vi "Teleop.vi"(10 "Match Info":T1={"Autonomous Elapsed Seconds"=0.0, "TeleOp Elapsed Seconds"=0.0, "Disabled Elapsed Seconds"=0.0, "Visited Autonomous"=FALSE, "Visited TeleOp"=FALSE, "Visited Disabled"=FALSE, "Autonomous Settings"={"Autonomous Style"=enum."Independent", "VI Refnum"=refnum}}, 11 "Call Context":T2) -> ()   [LabVIEW 2011]
doc: "This VI is called for each TeleOp packet received from the DS where the robot is not disabled. It is often used to read from the joysticks and update I/O or to update setpoints for timed control loops. It should complete and return within 20 milliseconds or it may miss DS packets."
uses:
  <vilib>/Rock Robotics/WPI/DriverStation/WPI_DriverStationDerivedRobotMode.ctl
  <vilib>/Rock Robotics/WPI/DriverStation/WPI_DriverStationMatch Info.ctl
  <vilib>/Rock Robotics/WPI/Relay/WPI_RelayValue.ctl
  <vilib>/Rock Robotics/WPI/DriverStation/DriverStationLCD/WPI_DriverStationLCDLCDLine.ctl
  Robot Global Data.vi
panel:
  in  "LDrive0":dbl
  in  "Rdrive0":dbl=0.9
  in  "Rdrive2":dbl=0.6
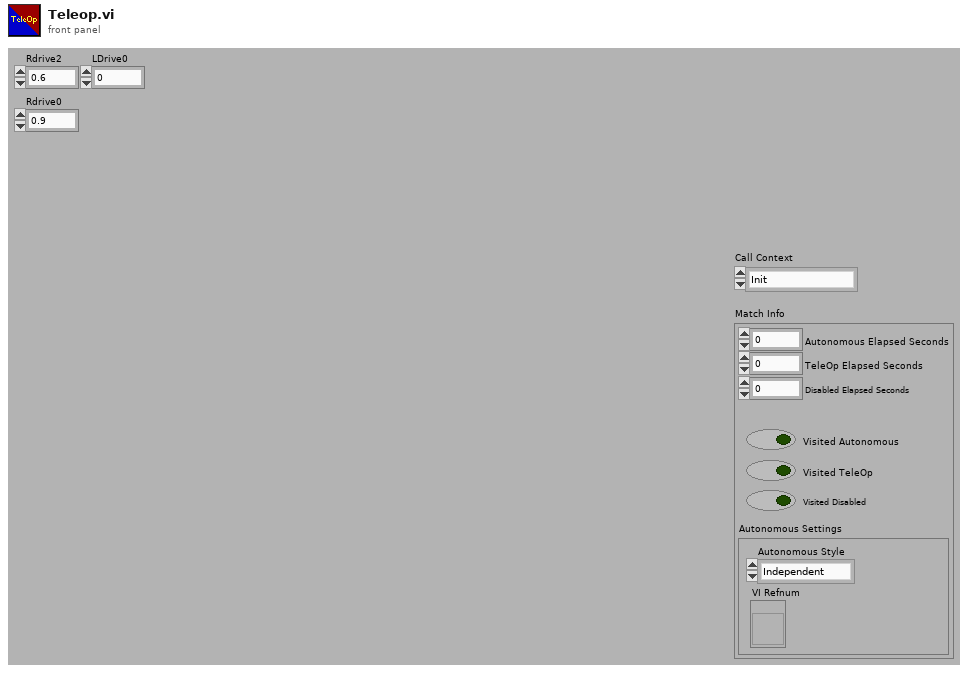
[diagram p1: front panel]
types:
  T1 = typedef "WPI_DriverStationMatch Info.ctl" = cluster{"Autonomous Elapsed Seconds":dbl, "TeleOp Elapsed Seconds":dbl, "Disabled Elapsed Seconds":dbl, "Visited Autonomous":bool, "Visited TeleOp":bool, "Visited Disabled":bool, "Autonomous Settings":cluster{"Autonomous Style":enum16{"Iterative", "Independent"}, "VI Refnum":refnum<vi>}}
  T2 = typedef "WPI_DriverStationDerivedRobotMode.ctl" = enum16{"Init", "Execute", "Stop"}
  T3 = typedef "WPI_RelayValue.ctl" = enum16{"Off", "On", "Forward", "Reverse"}
  T4 = typedef "WPI_JoystickDevRef.ctl" = cluster{"Device":T5}
  T5 = typedef "WPI_JoystickDeviceEnum.ctl" = enum16{"USB 1", "USB 2", "USB 3", "USB 4", "Kinect 1", "Kinect 2"}
  T6 = typedef "WPI_JoystickButtonState.ctl" = cluster{"Button 1":bool, "Button 2":bool, "Button 3":bool, "Button 4":bool, "Button 5":bool, "Button 6":bool, "Button 7":bool, "Button 8":bool, "Button 9":bool, "Button 10":bool, "Button 11":bool, "Button 12":bool}
  T7 = cluster{"axis 1 (x)":dbl, "axis 2 (y)":dbl, "axis 3 (throttle)":dbl, "axis 4":dbl, "axis 5":dbl, "axis 6":dbl}
  T8 = typedef "WPI_MotorControlDeviceRef.ctl" = cluster{"DeviceStatus":errorcluster, "Type":enum16{"PWM", "CAN"}, "PWM":cluster{"Digital Module":T9, "PWM Channel":T10, "DeadBand":T11}, "CAN":cluster{"Device Number":u8, "Control Mode":T12, "Semaphore":T13, "Max Vout":dbl}, "Invert":bool, "TransformRef":T14, "InvTransformRef":T14}
  T9 = typedef "FPGA_TypedefDigitalModule.ctl" = enum16{"Digital Module 1", "Digital Module 2"}
  T10 = typedef "FPGA_DIOPWMChannel.ctl" = enum8{"PWM 1", "PWM 2", "PWM 3", "PWM 4", "PWM 5", "PWM 6", "PWM 7", "PWM 8", "PWM 9", "PWM 10", "Invalid"}
  T11 = typedef "WPI_PWMDeadband.ctl" = cluster{"Name":string, "maxPositivePwm":i32, "minPositivePwm":i32, "centerPwm":i32, "maxNegativePwm":i32, "minNegativePwm":i32, "angularRange":u16}
  T12 = typedef "WPI_CANJaguar_ControlMode.ctl" = enum8{"Percent VBus", "Current", "Speed", "Position", "Voltage"}
  T13 = typedef "Semaphore RefNum" = refnum<k1>
  T14 = typedef "WPI_PWMTransform_ConPane.ctl" = refnum<vi>
  T15 = cluster{"Driver Station Digital Input (1-8)[0]":bool, "Driver Station Digital Input (1-8)[1]":bool, "Driver Station Digital Input (1-8)[2]":bool, "Driver Station Digital Input (1-8)[3]":bool, "Driver Station Digital Input (1-8)[4]":bool, "Driver Station Digital Input (1-8)[5]":bool, "Driver Station Digital Input (1-8)[6]":bool, "Driver Station Digital Input (1-8)[7]":bool, "Driver Station Digital Input (1-8)[8]":bool}
  T16 = typedef "WPI_RelayDevRef.ctl" = cluster{"DevStatus":errorcluster, "Relay Channel":T17, "Digital Module":T9, "Relay Direction":T18}
  T17 = typedef "FPGA_DIORelayChannel.ctl" = enum8{"Relay 1", "Relay 2", "Relay 3", "Relay 4", "Relay 5", "Relay 6", "Relay 7", "Relay 8", "Invalid"}
  T18 = typedef "WPI_RelayDirection.ctl" = enum16{"Both directions", "Forward only", "Reverse only"}
  T19 = typedef "WPI_DigitalInputDevRef.ctl" = cluster{"DevStatus":errorcluster, "DIO Channel":T20, "Digital Module":T9}
  T20 = typedef "FPGA_DIOChannel.ctl" = enum8{"DIO 1", "DIO 2", "DIO 3", "DIO 4", "DIO 5", "DIO 6", "DIO 7", "DIO 8", "DIO 9", "DIO 10", "DIO 11", "DIO 12", "DIO 13", "DIO 14", "Invalid"}
  T21 = typedef "WPI_EncoderDevRef.ctl" = cluster{"DevStatus":errorcluster, "EncoderIndex":T22, "CounterIndex":T23, "DistancePerCount":dbl, "Decoding Type":T24}
  T22 = typedef "FPGA_EncoderIdx.ctl" = enum8{"Enc 0", "Enc 1", "Enc 2", "Enc 3", "Invalid"}
  T23 = typedef "FPGA_CounterCtrSystemIndex.ctl" = enum8{"Ctr 0", "Ctr 1", "Ctr 2", "Ctr 3", "Ctr 4", "Ctr 5", "Ctr 6", "Ctr 7", "Invalid"}
  T24 = typedef "WPI_EncoderType.ctl" = enum16{"1x", "2x", "4x"}
  T25 = typedef "WPI_DriverStationLCDLCDLine.ctl" = enum16{"Main - Line 1", "User - Line 2", "User - Line 3", "User - Line 4", "User - Line 5", "User - Line 6"}
  T26 = typedef "WPI_ServoDeviceRef.ctl" = cluster{"DeviceStatus":errorcluster, "Digital Module":T9, "PWM Channel":T10, "DeadBand":T11}
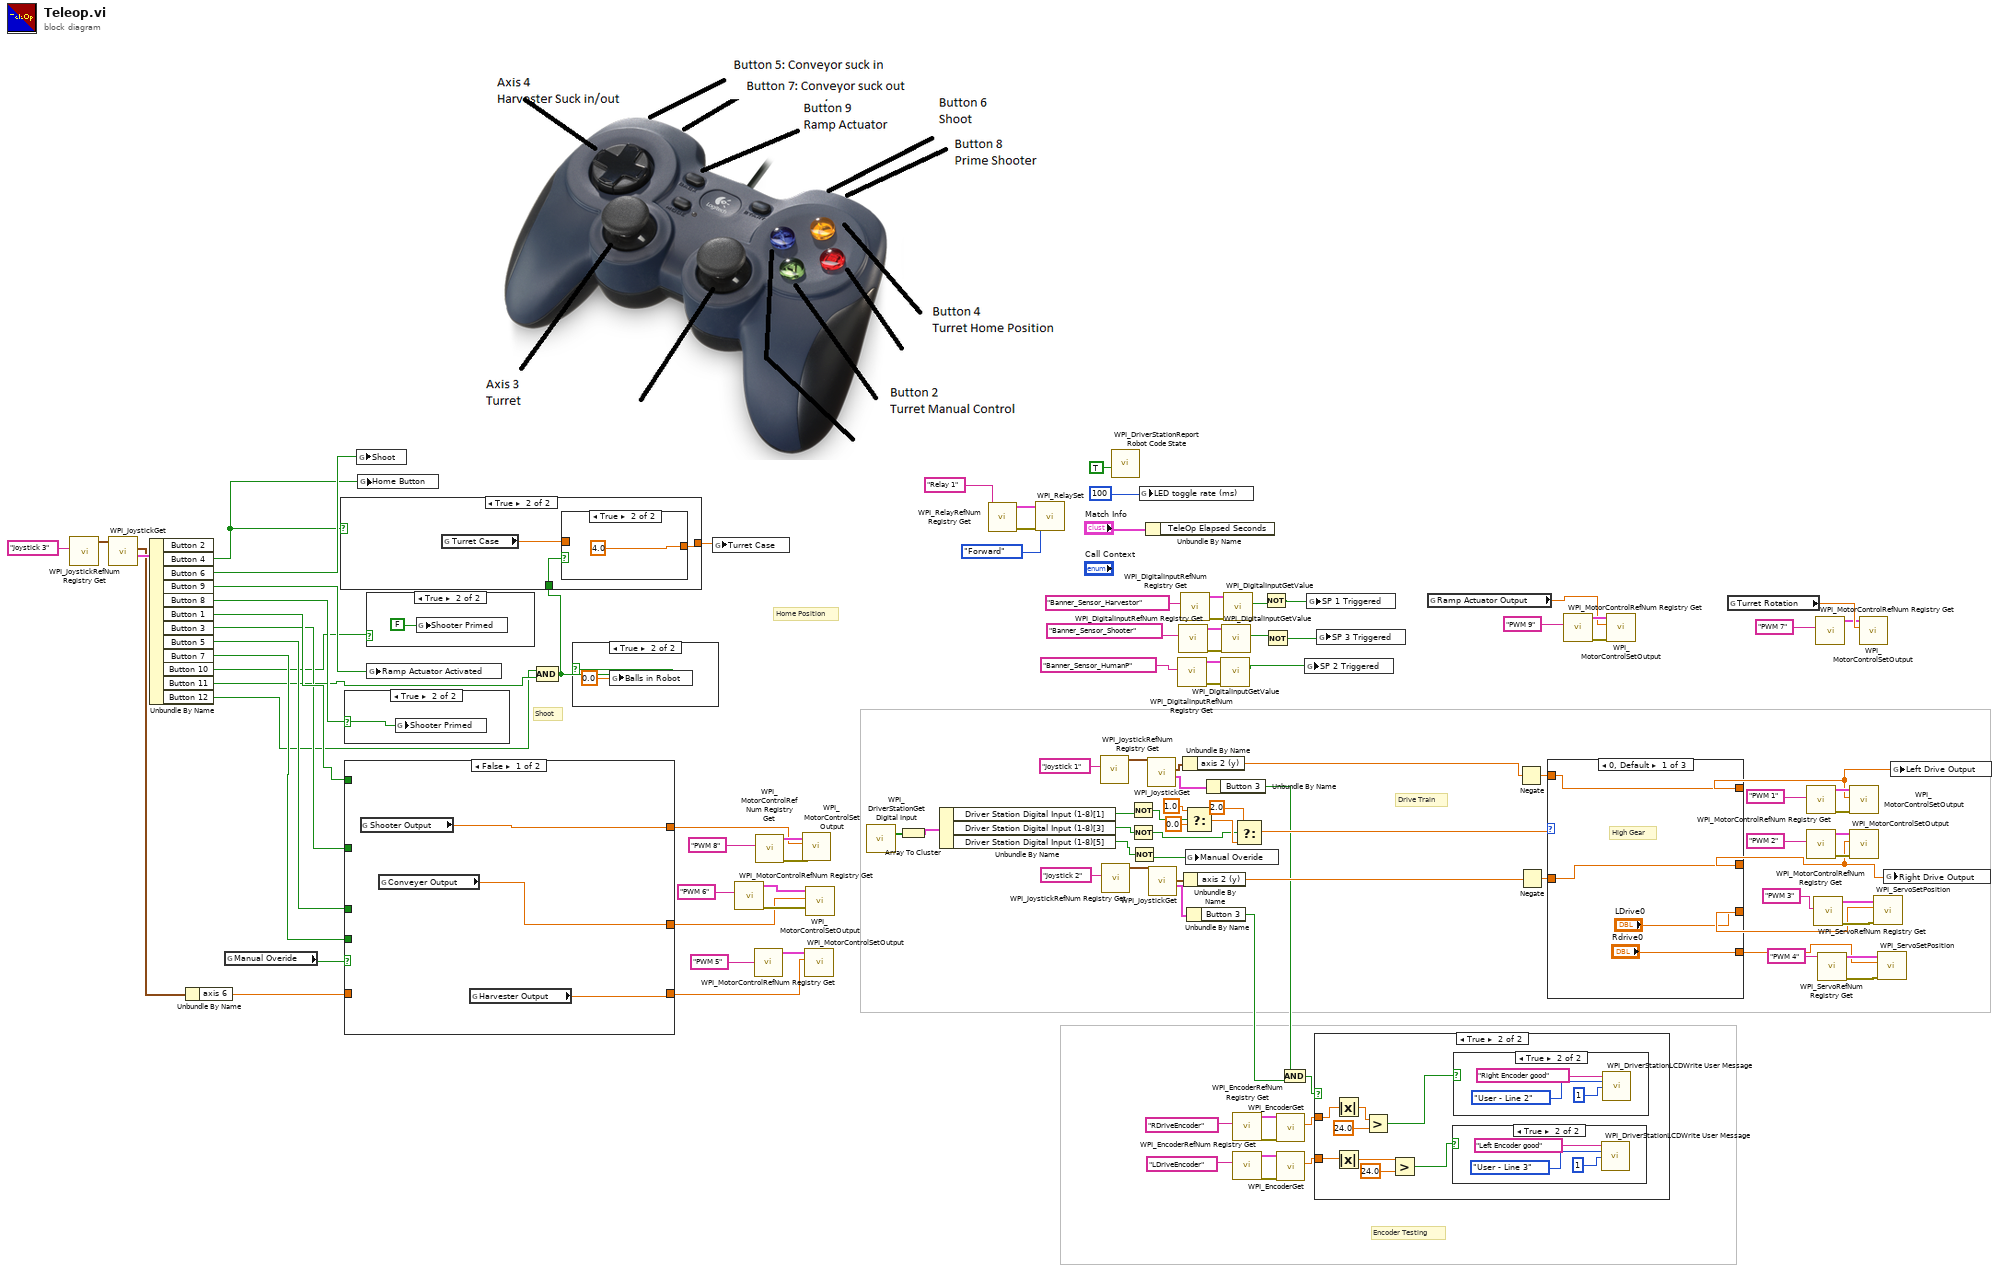
[diagram p0: block diagram]
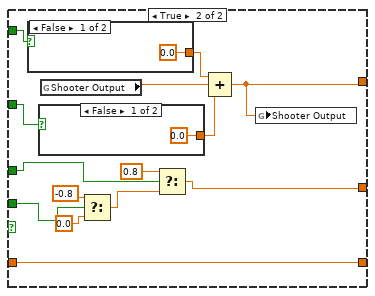
[diagram p7: hidden frame]
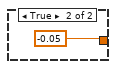
[diagram p8: hidden frame]
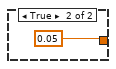
[diagram p9: hidden frame]
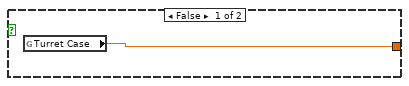
[diagram p11: hidden frame]
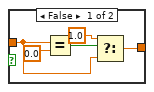
[diagram p12: hidden frame]
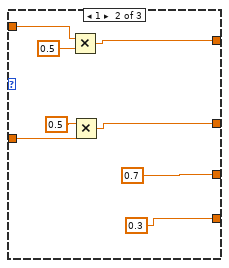
[diagram p13: hidden frame]
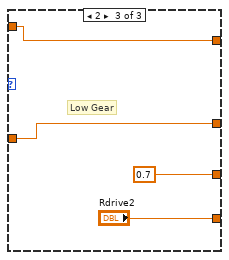
[diagram p14: hidden frame]
diagram:
  # "Encoder Testing"
  # "Shoot"
  # "Home Position"
  # "Drive Train"
  n1 = call <vilib>:"WPI_JoystickRefNum Registry Get.vi"("refnum name"="Joystick 3") -> ("JoystickDevRef"=w63:T4)  [unwired: 9 in, 1 out]
  n2 = call <vilib>:"WPI_JoystickGet.vi"("JoystickDevRef"=w63) -> ("Buttons"=w64:T6, "Axes"=w37:T7)  [unwired: 4 in, 1 out]
  n3 = Unbundle By Name(w64) -> ("Button 4"=w22:bool, "Button 6"=w62:bool, "Button 9"=w66:bool, "Button 8"=w38:bool, "Button 1"=w24:bool, "Button 3"=w23:bool, "Button 5"=w32:bool, "Button 7"=w31:bool, "Button 10"=w21:bool, "Button 11"=w20:bool, "Button 12"=w19:bool)  [unwired: 1 out]
  n4 = Unbundle By Name(w37) -> ("axis 6"=w17:dbl)
  n5 = global read "Robot Global Data.vi" "Manual Overide"() -> (w26:bool)
  n6 = case shown="True" w38 {
    selector: w38 -> [_ w111]
    frame False {
    }
    frame True {
      n7 = global write "Robot Global Data.vi" "Shooter Primed"(w111) -> ()
    }
  }
  n8 = case shown="False" w26 {
    tunnel: [w114 w116] -> w33
    tunnel: w24 -> [_ w121]
    tunnel: w23 -> [_ w120]
    tunnel: w32 -> [_ w123]
    tunnel: w31 -> [_ w124]
    tunnel: [w113 w122] -> w27
    tunnel: [w112 w115] -> w18
    tunnel: w17 -> [_ w115]
    frame False {
      n9 = global read "Robot Global Data.vi" "Shooter Output"() -> (w114:dbl)
      n10 = global read "Robot Global Data.vi" "Conveyer Output"() -> (w113:dbl)
      n11 = global read "Robot Global Data.vi" "Harvester Output"() -> (w112:dbl)
    }
    frame True {
      n12 = case shown="False" w121 {
        tunnel: [0.0 0.05] -> w119
        frame False {
        }
        frame True {
        }
      }
      n13 = case shown="False" w120 {
        tunnel: [0.0 -0.05] -> w118
        frame False {
        }
        frame True {
        }
      }
      n14 = global read "Robot Global Data.vi" "Shooter Output"() -> (w117:dbl)
      n15 = Select(t=-0.8, s=w124, f=0.0) -> (s? t:f=w128:dbl)
      n16 = Select(t=0.8, s=w123, f=w128) -> (s? t:f=w122:dbl)
      n17 = Compound Arithmetic op=ADD(w119, w117, w118) -> (w116:dbl)
      n18 = global write "Robot Global Data.vi" "Shooter Output"(w116) -> ()
    }
  }
  n19 = global write "Robot Global Data.vi" "Shoot"(w62) -> ()
  n20 = global write "Robot Global Data.vi" "Home Button"(w22) -> ()
  n21 = case shown="True" w21 {
    frame False {
    }
    frame True {
      n22 = global write "Robot Global Data.vi" "Shooter Primed"(FALSE ("Shooter Primed")) -> ()
    }
  }
  n23 = global write "Robot Global Data.vi" "Ramp Actuator Activated"(w66) -> ()
  n24 = Compound Arithmetic op=AND(w19, w20) -> (w16:bool)
  n25 = case shown="True" w22 {
    tunnel: [w134 w135] -> w15
    tunnel: w16 -> [_ w137]
    frame False {
      n26 = global read "Robot Global Data.vi" "Turret Case"() -> (w134:dbl)
    }
    frame True {
      n27 = global read "Robot Global Data.vi" "Turret Case"() -> (w136:dbl)
      n28 = case shown="True" w137 {
        tunnel: w136 -> [w139 _]
        tunnel: [w138 4.0 ("Turret Case")] -> w135
        frame False {
          n29 = Equal?(x=w139, y=0.0) -> (x = y?=w141:bool)
          n30 = Select(t=1.0, s=w141, f=w139) -> (s? t:f=w138:dbl)
        }
        frame True {
        }
      }
    }
  }
  n31 = case shown="True" w16 {
    frame False {
    }
    frame True {
      n32 = global write "Robot Global Data.vi" "Balls in Robot"(0.0 ("Balls in Robot")) -> ()
    }
  }
  n33 = global write "Robot Global Data.vi" "Turret Case"(w15) -> ()
  n34 = call <vilib>:"WPI_MotorControlRefNum Registry Get.vi"("refnum name"="PWM 6") -> ("error out"=w28:errorcluster, "MotorControlDevRef"=w29:T8)  [unwired: 9 in]
  n35 = call <vilib>:"WPI_MotorControlRefNum Registry Get.vi"("refnum name"="PWM 5") -> ("MotorControlDevRef"=w56:T8)  [unwired: 9 in, 1 out]
  n36 = call <vilib>:"WPI_MotorControlRefNum Registry Get.vi"("refnum name"="PWM 8") -> ("error out"=w40:errorcluster, "MotorControlDevRef"=w41:T8)  [unwired: 9 in]
  n37 = call <vilib>:"WPI_MotorControlSetOutput.vi"("error in (no error)"=w40, "Output"=w33, "MotorControlDevRef"=w41) -> ()  [unwired: 7 in, 2 out]
  n38 = call <vilib>:"WPI_MotorControlSetOutput.vi"("Output"=w18, "MotorControlDevRef"=w56) -> ()  [unwired: 8 in, 2 out]
  n39 = call <vilib>:"WPI_MotorControlSetOutput.vi"("error in (no error)"=w28, "Output"=w27, "MotorControlDevRef"=w29) -> ()  [unwired: 7 in, 2 out]
  n40 = call <vilib>:"WPI_DriverStationGet Digital Input.vi"() -> ("Driver Station Digital Input (1-8)"=w85:bool[])  [unwired: 11 in]
  n41 = Array To Cluster(array=w85) -> (cluster=w107:T15)
  n42 = Unbundle By Name(w107) -> ("Driver Station Digital Input (1-8)[1]"=w88:bool, "Driver Station Digital Input (1-8)[3]"=w87:bool, "Driver Station Digital Input (1-8)[5]"=w34:bool)
  n43 = call <vilib>:"WPI_RelayRefNum Registry Get.vi"("refnum name"="Relay 1") -> ("error out"=w60:errorcluster, "RelayDevRef"=w61:T16)  [unwired: 9 in]
  n44 = call <vilib>:"WPI_RelaySet.vi"("error in (no error)"=w60, "RelayValue"=WPI_RelayValue."Forward", "RelayDevRef"=w61) -> ()  [unwired: 7 in, 2 out]
  n45 = call <vilib>:"WPI_JoystickRefNum Registry Get.vi"("refnum name"="Joystick 1") -> ("JoystickDevRef"=w100:T4)  [unwired: 9 in, 1 out]
  n46 = call <vilib>:"WPI_JoystickRefNum Registry Get.vi"("refnum name"="Joystick 2") -> ("JoystickDevRef"=w98:T4)  [unwired: 9 in, 1 out]
  n47 = call <vilib>:"WPI_DriverStationReport Robot Code State.vi"("TeleOp"=TRUE ("Autonomous")) -> ()  [unwired: 10 in, 1 out]
  n48 = Not(x=w88) -> (.not. x?=w86:bool)
  n49 = Not(x=w87) -> (.not. x?=w36:bool)
  n50 = Not(x=w34) -> (.not. x?=w35:bool)
  n51 = global write "Robot Global Data.vi" "LED toggle rate (ms)"(u32 100 ("LED ms toggle rate")) -> ()
  n52 = Unbundle By Name("Match Info") -> ()  [unwired: 1 out]
  n53 = call <vilib>:"WPI_JoystickGet.vi"("JoystickDevRef"=w100) -> ("Buttons"=w12:T6, "Axes"=w13:T7)  [unwired: 4 in, 1 out]
  n54 = call <vilib>:"WPI_JoystickGet.vi"("JoystickDevRef"=w98) -> ("Buttons"=w14:T6, "Axes"=w99:T7)  [unwired: 4 in, 1 out]
  n55 = call <vilib>:"WPI_DigitalInputRefNum Registry Get.vi"("refnum name"="Banner_Sensor_HumanP") -> ("error out"=w51:errorcluster, "DigitalInputDevRef"=w50:T19)  [unwired: 9 in]
  n56 = call <vilib>:"WPI_DigitalInputRefNum Registry Get.vi"("refnum name"="Banner_Sensor_Shooter") -> ("error out"=w52:errorcluster, "DigitalInputDevRef"=w53:T19)  [unwired: 9 in]
  n57 = call <vilib>:"WPI_DigitalInputRefNum Registry Get.vi"("refnum name"="Banner_Sensor_Harvestor") -> ("error out"=w55:errorcluster, "DigitalInputDevRef"=w54:T19)  [unwired: 9 in]
  n58 = Unbundle By Name(w13) -> ("axis 2 (y)"=w84:dbl)
  n59 = Unbundle By Name(w99) -> ("axis 2 (y)"=w82:dbl)
  n60 = Select(t=1.0, s=w86, f=0.0 ("t")) -> (s? t:f=w104:dbl)
  n61 = global write "Robot Global Data.vi" "Manual Overide"(w35) -> ()
  n62 = Unbundle By Name(w14) -> ("Button 3"=w10:bool)
  n63 = Unbundle By Name(w12) -> ("Button 3"=w11:bool)
  n64 = call <vilib>:"WPI_DigitalInputGetValue.vi"("error in (no error)"=w51, "DigitalInputDevRef"=w50) -> ("Value"=w46:bool)  [unwired: 7 in, 2 out]
  n65 = call <vilib>:"WPI_DigitalInputGetValue.vi"("error in (no error)"=w52, "DigitalInputDevRef"=w53) -> ("Value"=w45:bool)  [unwired: 7 in, 2 out]
  n66 = call <vilib>:"WPI_DigitalInputGetValue.vi"("error in (no error)"=w55, "DigitalInputDevRef"=w54) -> ("Value"=w43:bool)  [unwired: 7 in, 2 out]
  n67 = call <vilib>:"WPI_EncoderRefNum Registry Get.vi"("refnum name"="RDriveEncoder") -> ("error out"=w6:errorcluster, "EncoderDevRef"=w7:T21)  [unwired: 9 in]
  n68 = call <vilib>:"WPI_EncoderRefNum Registry Get.vi"("refnum name"="LDriveEncoder") -> ("error out"=w5:errorcluster, "EncoderDevRef"=w4:T21)  [unwired: 9 in]
  n69 = Select(t=2.0, s=w36, f=w104) -> (s? t:f=w102:dbl)
  n70 = Not(x=w43) -> (.not. x?=w42:bool)
  n71 = Not(x=w45) -> (.not. x?=w44:bool)
  n72 = call <vilib>:"WPI_EncoderGet.vi"("error in (no error)"=w6, "EncoderDevRef"=w7) -> ("Distance"=w2:dbl)  [unwired: 4 in, 5 out]
  n73 = call <vilib>:"WPI_EncoderGet.vi"("error in (no error)"=w5, "EncoderDevRef"=w4) -> ("Distance"=w1:dbl)  [unwired: 4 in, 5 out]
  n74 = And(x=w11, y=w10) -> (x .and. y?=w9:bool)
  n75 = global write "Robot Global Data.vi" "SP 2 Triggered"(w46) -> ()
  n76 = global write "Robot Global Data.vi" "SP 1 Triggered"(w42) -> ()
  n77 = case shown="True" w9 {
    tunnel: w2 -> [_ w147]
    tunnel: w1 -> [_ w146]
    frame False {
    }
    frame True {
      n78 = Absolute Value(x=w147) -> (abs(x)=w148:dbl)
      n79 = Absolute Value(x=w146) -> (abs(x)=w145:dbl)
      n80 = Greater?(x=w148, y=24.0) -> (0:w151:bool)
      n81 = Greater?(x=w145, y=24.0) -> (0:w149:bool)
      n82 = case shown="True" w149 {
        frame False {
        }
        frame True {
          n83 = call <vilib>:"WPI_DriverStationLCDWrite User Message.vi"("line text"="Left Encoder good", "line"=WPI_DriverStationLCDLCDLine."User - Line 3", "starting column"=i8 1) -> ()  [unwired: 2 in, 11 out]
        }
      }
      n84 = case shown="True" w151 {
        frame False {
        }
        frame True {
          n85 = call <vilib>:"WPI_DriverStationLCDWrite User Message.vi"("line text"="Right Encoder good", "line"=WPI_DriverStationLCDLCDLine."User - Line 2", "starting column"=i8 1) -> ()  [unwired: 2 in, 11 out]
        }
      }
    }
  }
  n86 = global write "Robot Global Data.vi" "SP 3 Triggered"(w44) -> ()
  n87 = global read "Robot Global Data.vi" "Ramp Actuator Output"() -> (w25:dbl)
  n88 = Negate(x=w84) -> (-x=w83:dbl)
  n89 = Negate(x=w82) -> (-x=w81:dbl)
  n90 = case shown="0, Default" w102 {
    tunnel: w81 -> [w162 w167 w174]
    tunnel: [w162 w168 w174] -> w73
    tunnel: [w161 w169 w173] -> w74
    tunnel: ["LDrive0" 0.7 0.7] -> w90
    tunnel: ["Rdrive0" 0.3 ("LeftShifter_Pos") "Rdrive2"] -> w89
    tunnel: w83 -> [w161 w165 w173]
    frame 0, Default {
      # "High Gear"
    }
    frame 1 {
      n91 = Multiply(x=w165, y=0.5) -> (x*y=w169:dbl)
      n92 = Multiply(x=0.5 ("y"), y=w167) -> (x*y=w168:dbl)
    }
    frame 2 {
      # "Low Gear"
    }
  }
  n93 = call <vilib>:"WPI_MotorControlRefNum Registry Get.vi"("refnum name"="PWM 9") -> ("error out"=w71:errorcluster, "MotorControlDevRef"=w70:T8)  [unwired: 9 in]
  n94 = call <vilib>:"WPI_MotorControlSetOutput.vi"("error in (no error)"=w71, "Output"=w25, "MotorControlDevRef"=w70) -> ()  [unwired: 7 in, 2 out]
  n95 = global read "Robot Global Data.vi" "Turret Rotation"() -> (w69:dbl)
  n96 = call <vilib>:"WPI_MotorControlRefNum Registry Get.vi"("refnum name"="PWM 1") -> ("error out"=w78:errorcluster, "MotorControlDevRef"=w80:T8)  [unwired: 9 in]
  n97 = call <vilib>:"WPI_MotorControlRefNum Registry Get.vi"("refnum name"="PWM 2") -> ("error out"=w77:errorcluster, "MotorControlDevRef"=w76:T8)  [unwired: 9 in]
  n98 = call <vilib>:"WPI_ServoRefNum Registry Get.vi"("refnum name"="PWM 3") -> ("error out"=w94:errorcluster, "ServoDeviceRef"=w95:T26)  [unwired: 9 in]
  n99 = call <vilib>:"WPI_MotorControlRefNum Registry Get.vi"("refnum name"="PWM 7") -> ("MotorControlDevRef"=w67:T8)  [unwired: 9 in, 1 out]
  n100 = call <vilib>:"WPI_ServoRefNum Registry Get.vi"("refnum name"="PWM 4") -> ("error out"=w93:errorcluster, "ServoDeviceRef"=w92:T26)  [unwired: 9 in]
  n101 = call <vilib>:"WPI_MotorControlSetOutput.vi"("error in (no error)"=w78, "Output"=w74, "MotorControlDevRef"=w80) -> ()  [unwired: 7 in, 2 out]
  n102 = call <vilib>:"WPI_MotorControlSetOutput.vi"("error in (no error)"=w77, "Output"=w73, "MotorControlDevRef"=w76) -> ()  [unwired: 7 in, 2 out]
  n103 = call <vilib>:"WPI_MotorControlSetOutput.vi"("Output"=w69, "MotorControlDevRef"=w67) -> ()  [unwired: 8 in, 2 out]
  n104 = call <vilib>:"WPI_ServoSetPosition.vi"("error in (no error)"=w94, "Position"=w90, "ServoDeviceRef"=w95) -> ()  [unwired: 7 in, 2 out]
  n105 = call <vilib>:"WPI_ServoSetPosition.vi"("error in (no error)"=w93, "Position"=w89, "ServoDeviceRef"=w92) -> ()  [unwired: 7 in, 2 out]
  n106 = global write "Robot Global Data.vi" "Right Drive Output"(w73) -> ()
  n107 = global write "Robot Global Data.vi" "Left Drive Output"(w74) -> ()
